vi "Rebuild Score Data From Files.vi"(11 "Score Files Directory":path) -> ()   [LabVIEW 2013]
uses:
  <vilib>/Utility/miscctls.llb/LVDateTimeRec.ctl
  ScoreEntry.ctl
panel:
  out "Progress":dbl(slide) scale=0.0..1.0
  out "Array":cluster{"Name":string, "Value":string}[](array[cluster])
  out "Bad":bool
  out "Round":i32
  out "GUID":i32
  out "Timestamp":timestamp
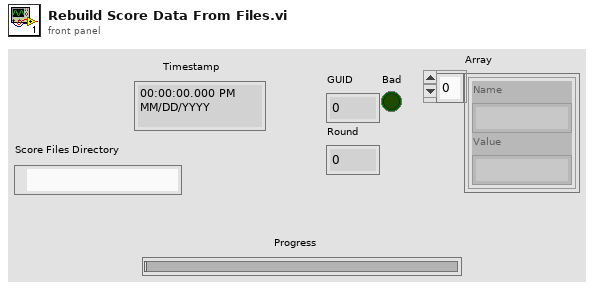
[diagram p1: front panel]
types:
  T1 = typedef "ScoreEntry.ctl" = cluster{"Elements":cluster{"Name":string, "Value":string}[], "Score":dbl}
  T2 = typedef "LVDateTimeRec.ctl" = cluster{"fractional second":dbl, "second":i32, "minute":i32, "hour":i32, "day of month":i32, "month":i32, "year":i32, "day of week":i32, "day of year":i32, "DST":i32}
  T3 = enum16{"open", "replace", "create", "open or create", "replace or create", "replace or create with confirmation"}
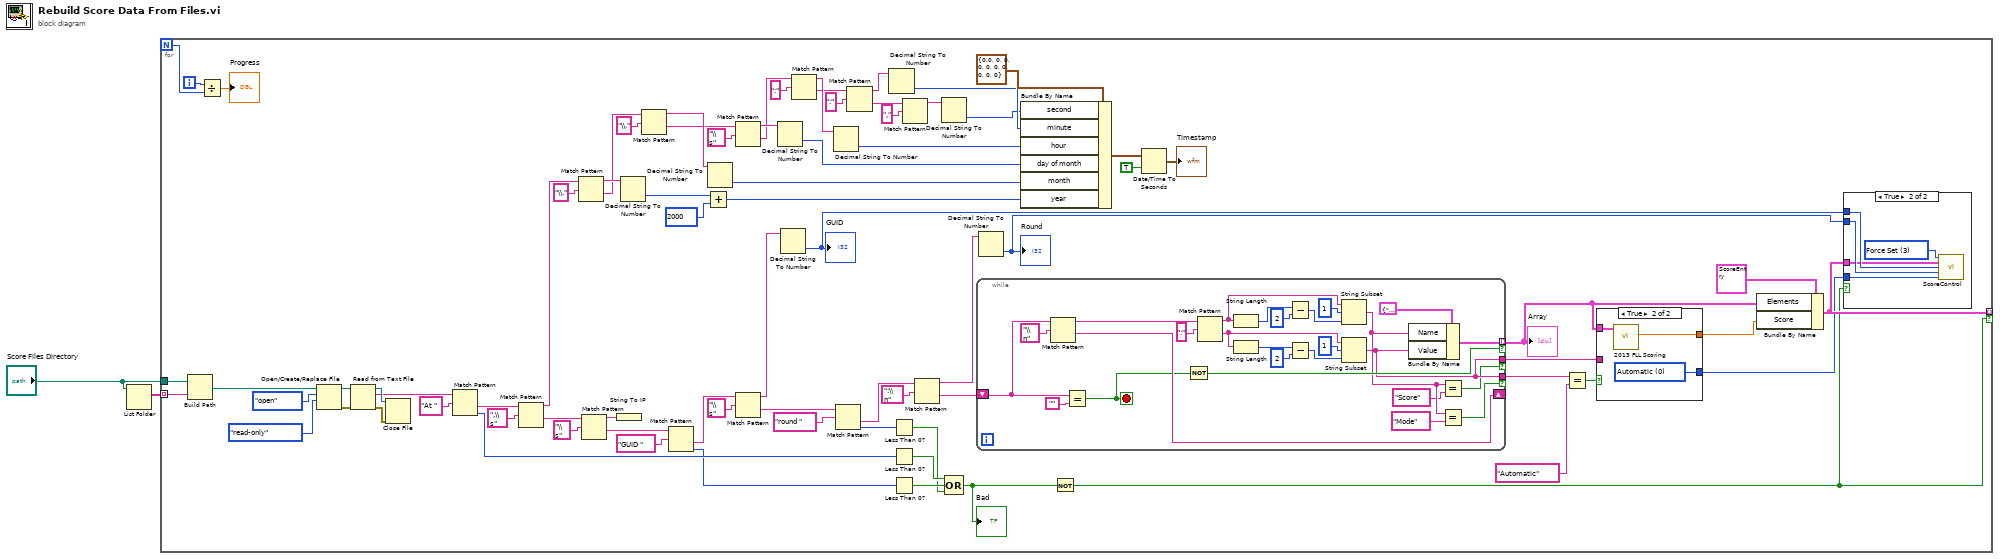
[diagram p0: block diagram]
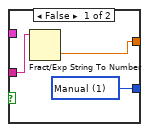
[diagram p3: hidden frame]
diagram:
  n1 = List Folder(path="Score Files Directory") -> (filenames=w2:string[])  [unwired: 3 in, 3 out]
  n2 = for {
    N -> [w18]
    tunnel: w2 -> [w80] mode=indexing
    tunnel: "Score Files Directory" -> [w81]
    tunnel: [w7] -> _ mode=indexing if=w6
    i -> [w17]
    n3 = Build Path(base path=w81, name or relative path=w80) -> (appended path=w79:path)
    n4 = Divide(x=w17, y=w18) -> (x/y=→"Progress":dbl)
    n5 = Open/Create/Replace File(file path (use dialog)=w79, operation (0:open)=T3."open", access (0:read/write)=enum16{"read/write", "read-only", "write-only"}."read-only") -> (refnum out=w76:refnum<file>, error out=w75:errorcluster)  [unwired: 3 in, 1 out]
    n6 = Read from Text File(file (use dialog)=w76, error in=w75) -> (refnum out=w74:refnum<file>, text=w72:string, error out=w73:errorcluster)  [unwired: 2 in, 1 out]
    n7 = Close File(refnum=w74, error in=w73) -> ()  [unwired: 2 out]
    n8 = Match Pattern(string=w72, regular expression="At ") -> (after substring=w70:string, offset past match=w26:i32)  [unwired: 1 in, 2 out]
    n9 = Match Pattern(string=w70, regular expression=",\\s") -> (before substring=w66:string, after substring=w38:string)  [unwired: 1 in, 2 out]
    n10 = Match Pattern(string=w66, regular expression="\\.") -> (before substring=w64:string, after substring=w62:string)  [unwired: 1 in, 2 out]
    n11 = Match Pattern(string=w38, regular expression="\\s") -> (before substring=w36:string, after substring=w35:string)  [unwired: 1 in, 2 out]
    n12 = String To IP(1:w36) -> ()  [unwired: 1 out]
    n13 = Decimal String To Number(string=w64) -> (number=w41:i32)  [unwired: 2 in, 1 out]
    n14 = Match Pattern(string=w62, regular expression="\\.") -> (before substring=w61:string, after substring=w57:string)  [unwired: 1 in, 2 out]
    n15 = Match Pattern(string=w35, regular expression="GUID ") -> (after substring=w33:string, offset past match=w25:i32)  [unwired: 1 in, 2 out]
    n16 = Add(x=w41, y=2000) -> (x+y=w39:i32)
    n17 = Decimal String To Number(string=w61) -> (number=w60:i32)  [unwired: 2 in, 1 out]
    n18 = Match Pattern(string=w57, regular expression="\\s") -> (before substring=w59:string, after substring=w55:string)  [unwired: 1 in, 2 out]
    n19 = Match Pattern(string=w33, regular expression="\\s") -> (before substring=w31:string, after substring=w30:string)  [unwired: 1 in, 2 out]
    n20 = Decimal String To Number(string=w59) -> (number=w56:i32)  [unwired: 2 in, 1 out]
    n21 = Decimal String To Number(string=w31) -> (number=w5:i32)  [unwired: 2 in, 1 out]
    "GUID" <- w5
    n22 = Match Pattern(string=w55, regular expression=":") -> (before substring=w53:string, after substring=w50:string)  [unwired: 1 in, 2 out]
    n23 = Decimal String To Number(string=w53) -> (number=w52:i32)  [unwired: 2 in, 1 out]
    n24 = Match Pattern(string=w30, regular expression="round ") -> (after substring=w28:string, offset past match=w24:i32)  [unwired: 1 in, 2 out]
    n25 = Match Pattern(string=w50, regular expression=":") -> (before substring=w49:string, after substring=w47:string)  [unwired: 1 in, 2 out]
    n26 = Decimal String To Number(string=w49) -> (number=w48:i32)  [unwired: 2 in, 1 out]
    n27 = Less Than 0?(x=w24) -> (x < 0?=w21:bool)
    n28 = Less Than 0?(x=w26) -> (x < 0?=w23:bool)
    n29 = Less Than 0?(x=w25) -> (x < 0?=w22:bool)
    n30 = Match Pattern(string=w47, regular expression=",") -> (before substring=w45:string)  [unwired: 1 in, 3 out]
    n31 = Match Pattern(string=w28, regular expression=":\\n") -> (before substring=w27:string, after substring=w19:string)  [unwired: 1 in, 2 out]
    n32 = Decimal String To Number(string=w45) -> (number=w44:i32)  [unwired: 2 in, 1 out]
    n33 = Compound Arithmetic op=OR(w23, w22, w21) -> (w8:bool)
    "Bad" <- w8
    n34 = while {
      shift-right: [w117] -> _
      shift-left: w19 -> [w116]
      tunnel: [w103] -> w14 mode=indexing if=w101
      tunnel: [w94] -> w12 if=w97
      tunnel: [w94] -> w9 if=w93
      stop <- w102 stop-if-true
      n35 = Match Pattern(string=w116, regular expression="\\n") -> (before substring=w114:string, after substring=w117:string)  [unwired: 1 in, 2 out]
      n36 = Equal?(x=w116, y="") -> (x = y?=w102:bool)
      n37 = Not(x=w102) -> (.not. x?=w101:bool)
      n38 = Match Pattern(string=w114, regular expression=":" ("search string/char (-)")) -> (before substring=w111:string, after substring=w100:string)  [unwired: 1 in, 2 out]
      n39 = String Length(string=w111) -> (length=w110:i32)
      n40 = String Length(string=w100) -> (length=w106:i32)
      n41 = Subtract(x=w110, y=2) -> (x-y=w108:i32)
      n42 = Subtract(x=w106, y=2) -> (x-y=w99:i32)
      n43 = String Subset(string=w111, offset (0)=1, length (rest)=w108) -> (substring=w96:string)
      n44 = String Subset(string=w100, offset (0)=1, length (rest)=w99) -> (substring=w94:string)
      n45 = Bundle By Name(cluster=cluster{"Name":string, "Value":string} {"Name"="", "Value"=""}, "Name"=w96, "Value"=w94) -> (w103:cluster{"Name":string, "Value":string})
      n46 = Equal?(x=w96, y="Score") -> (x = y?=w93:bool)
      n47 = Equal?(x=w96, y="Mode") -> (x = y?=w97:bool)
    }
    "Array" <- w14
    n48 = Decimal String To Number(string=w27) -> (number=w4:i32)  [unwired: 2 in, 1 out]
    "Round" <- w4
    n49 = Bundle By Name(cluster=T2 {"fractional second"=0.0, "second"=0, "minute"=0, "hour"=0, "day of month"=0, "month"=0, "year"=0, "day of week"=0, "day of year"=0, "DST"=0} ("date time rec"), "second"=w44, "minute"=w48, "hour"=w52, "day of month"=w56, "month"=w60, "year"=w39) -> (w67:T2)
    n50 = Not(x=w8) -> (.not. x?=w6:bool)
    n51 = Date/Time To Seconds(1:TRUE ("is UTC (F)"), 2:w67) -> (0:→"Timestamp":timestamp)
    n52 = Equal?(x=w12, y="Automatic") -> (x = y?=w10:bool)
    n53 = case shown="True" w10 {
      tunnel: w14 -> [_ w92]
      tunnel: [w88 w91] -> w13
      tunnel: w9 -> [w89 _]
      tunnel: [w87 w90] -> w3
      frame False {
        w87 = u16 1 items=["Automatic", "Manual"] ("Score Mode Selector")
        n54 = Fract/Exp String To Number(string=w89) -> (number=w88:dbl)  [unwired: 3 in, 1 out]
      }
      frame True {
        w90 = u16 0 items=["Automatic", "Manual"] ("Score Mode Selector")
        n55 = call "2013 FLL Scoring.vi"("Array"=w92) -> ("Total Score"=w91:dbl)  [unwired: 9 in, 1 out]
      }
    }
    n56 = Bundle By Name(cluster=T1 {"Elements"=[{"Name"="CO2 Balls Touching/Within Reservoir Model", "Value"="-1"}, {"Name"="Money Ball Touching/Within Reservoir Model", "Value"="-1"}, {"Name"="3+ Red/White Citizens in Pink Grid Area", "Value"="-1"}, {"Name"="# Upright Levee Blocks touching ONLY GREEN shores", "Value"="-1"}, {"Name"="# Upright Levee Blocks Touching any RED shore", "Value"="-1"}, {"Name"="Levee Test was Performed", "Value"="-1"}, {"Name"="Levee Test Wheel Blocked by NonLevee", "Value"="-1"}, {"Name"="Flood Barrier in Up Position", "Value"="-1"}, {"Name"="Both Yellow Arrows Aligned", "Value"="-1"}, {"Name"="Team Robot Touching Only Yellow Grid Area", "Value"="-1"}, {"Name"="Both Insulation Touching Green Grid Area", "Value"="-1"}, {"Name"="Bicycle Touching Green Grid Area", "Value"="-1"}, {"Name"="Computer Touching Green Grid Area", "Value"="-1"}, {"Name"="House in Up Position", "Value"="-1"}, {"Name"="House Window Showing Black", "Value"="-1"}, {"Name"="House Window All The Way Open", "Value"="-1"}, {"Name"="3+ Black/White Scientists Touching Research Area", "Value"="-1"}, {"Name"="Money Ball Touching/Within Research Area Model", "Value"="-1"}, {"Name"="Polar Bear Touching/Within Research Area Model", "Value"="-1"}, {"Name"="Polar Bear Orientation (Sleeping/Upright)", "Value"="-1"}, {"Name"="Ice Core Pulled From Its Hole", "Value"="-1"}, {"Name"="Ice Buoy Upright and Within/Touching Research Area Model", "Value"="-1"}, {"Name"="Drilling Machine Touching/Within Research Area Model", "Value"="-1"}, {"Name"="Drill Assembly Completely Vertical", "Value"="-1"}, {"Name"="Team Robot Touching/Within Research Area Model", "Value"="-1"}, {"Name"="3+ Blue/Gray Leaders Touching Green Mountain/City Area", "Value"="-1"}, {"Name"="Ice Core in Base Area", "Value"="-1"}, {"Name"="Snowmobile Touching/Within Research Area Model", "Value"="-1"}], "Score"=0.0} ("Full Score Entry"), "Elements"=w14, "Score"=w13) -> (w7:T1)
    n57 = case shown="True" w6 {
      tunnel: w5 -> [_ w85]
      tunnel: w4 -> [_ w84]
      tunnel: w7 -> [_ w83]
      tunnel: w3 -> [_ w82]
      frame False {
      }
      frame True {
        w86 = u16 3 items=["Get All", "Set", "Reset All", "Force Set", "Force Set All"] ("Get/Set Mode Selector")
        n58 = call "ScoreControl.vi"("Get/Set Mode Selector"=w86, "Full Score Entry"=w83, "GUID"=w85, "Round Number"=w84, "Score Mode Selector"=w82) -> ()  [unwired: 9 in, 2 out]
      }
    }
  }
